vi "Relative Move.vi"(6 "Timeout, s":dbl=10.0 format="%#_13g", 8 "error in (no error)":errorcluster, 9 "Axis (1..4)":u16(ring)=1 items=["X"=1, "Y"=2, "Z"=3, "Rotary"=4], 10 "Relative Move, counts":i32, 11 "VISA resource name":refnum<visa-resource-name>) -> (0 "error out":errorcluster, 1 "current position, counts":i32, 3 "VISA resource out":refnum<visa-resource-name>)   [LabVIEW 2017]
doc: "Relative move VI appropriate for short moves, < 5 seconds"
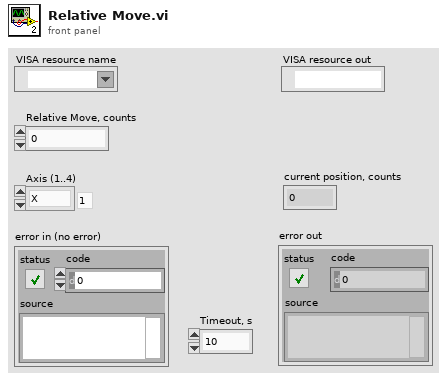
[diagram p1: front panel]
types:
  T1 = enum16{"Cmd-Response", "Write Only", "Read Only"}
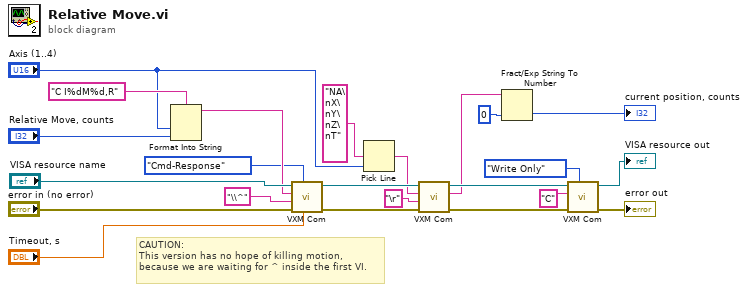
[diagram p0: block diagram]
diagram:
  # "CAUTION:\nThis version has no hope of killing motion,\nbecause we are waiting for ^ inside the first VI."
  n1 = Format Into String(format string="C I%dM%d,R", "Axis (1..4)", "Relative Move, counts") -> (resulting string=w20:string)  [unwired: 2 in, 1 out]
  n2 = call "VXM Com.vi"("Timeout, s"="Timeout, s", "Operation"=T1."Cmd-Response", "error in (no error)"="error in (no error)", "Termination String ('/' codes)"="\\^", "Write Buffer ('/' codes)"=w20, "VISA resource name"="VISA resource name") -> ("error out"=w13:errorcluster, "VISA resource out"=w16:refnum<visa-resource-name>)  [unwired: 3 in, 1 out]
  n3 = Pick Line(multi-line string="NA\nX\nY\nZ\nT", line index="Axis (1..4)") -> (output string=w7:string)  [unwired: 1 in]
  n4 = call "VXM Com.vi"("error in (no error)"=w13, "Termination String ('/' codes)"="\r", "Write Buffer ('/' codes)"=w7, "VISA resource name"=w16) -> ("error out"=w15:errorcluster, "Response String ('/' codes)"=w11:string, "VISA resource out"=w14:refnum<visa-resource-name>)  [unwired: 5 in]
  n5 = Fract/Exp String To Number(string=w11, default (0 dbl)=0 ("default (0 DBL)")) -> (number=→"current position, counts":i32)  [unwired: 2 in, 1 out]
  n6 = call "VXM Com.vi"("Operation"=T1."Write Only", "error in (no error)"=w15, "Write Buffer ('/' codes)"="C" ("Write Buffer"), "VISA resource name"=w14) -> ("error out"=→"error out":errorcluster, "VISA resource out"=→"VISA resource out":refnum<visa-resource-name>)  [unwired: 5 in, 1 out]
